vi "Main Page.vi"(8 "error in (no error)":errorcluster, 11 "Node Ptr":T1 format="%.0x") -> (0 "error out":errorcluster)   [LabVIEW 2016, in "UDP Sender System Explorer.lvlib"]
uses:
  UDP Sender System Explorer.lvlib
  <vilib>/NI Veristand/Custom Device API/Custom Device Item Ref.ctl
  Shared/Constants.vi
  <vilib>/NI Veristand/Custom Device API/Get Item Property (String).vi
  <vilib>/NI Veristand/Custom Device API/Get Item Property (U16).vi
  <vilib>/NI Veristand/Custom Device API/Set Item Property (String).vi
  <vilib>/NI Veristand/Custom Device API/Set Item Property (U16).vi
  <vilib>/NI Veristand/Custom Device API/Custom Device API.lvlib
  Shared/UDP Sender Shared.lvlib
panel:
  out "Channels to Send":i32(listbox)
  in  "Destination Port":u16
  in  "Destination IP":string
  in  "Header":cluster{"Section Name":string}={"Section Name"="Custom Device Item Settings"}
  in  "Description":string
  in  "Name":string
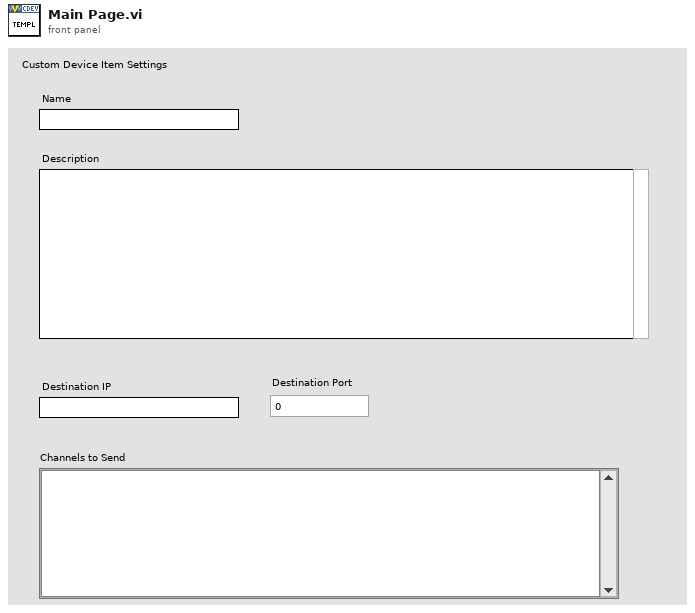
[diagram p1: front panel]
types:
  T1 = typedef "Custom Device API.lvlib/Custom Device Item Ref.ctl" = u64
  T2 = typedef "Custom Device API.lvlib/Custom Device Item Info.ctl" = cluster{"Name":string, "Is Channel":bool, "GUID":string, "Is Waveform":bool}
  T3 = typedef "Custom Device API.lvlib/Custom Device Commands.ctl" = enum16{"Default", "Item renamed", "Shutdown", "Dynamic button pressed"}
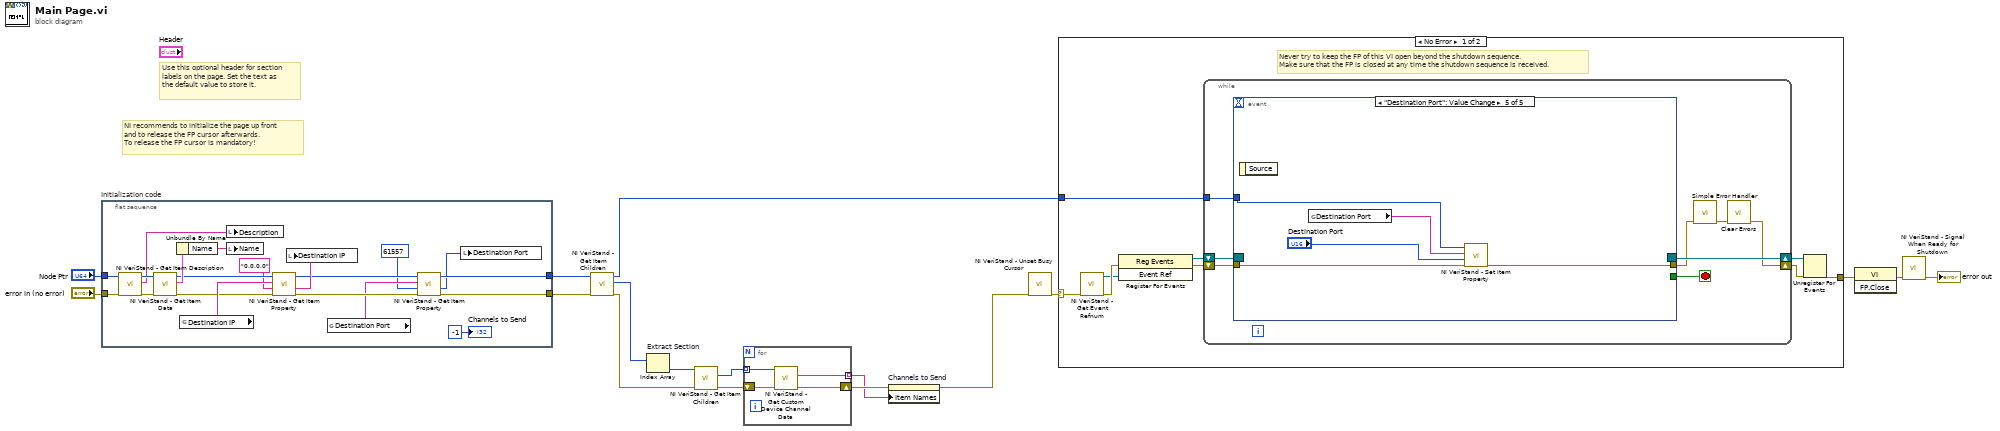
[diagram p0: block diagram]
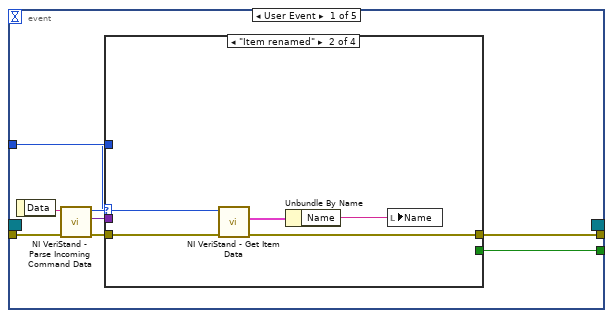
[diagram p2: hidden frame]
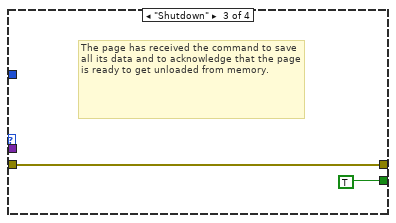
[diagram p4: hidden frame]
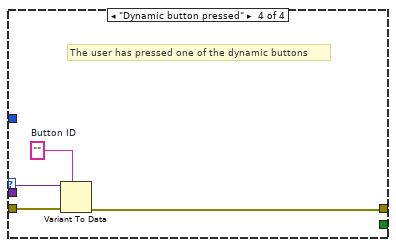
[diagram p5: hidden frame]
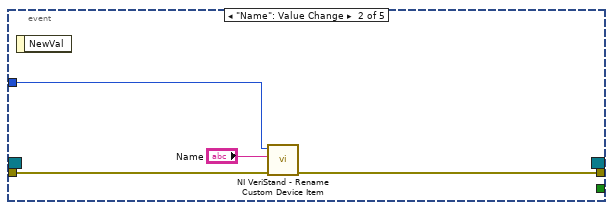
[diagram p6: hidden frame]
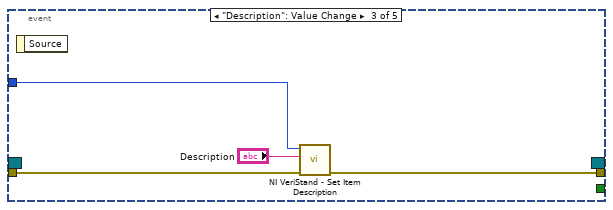
[diagram p7: hidden frame]
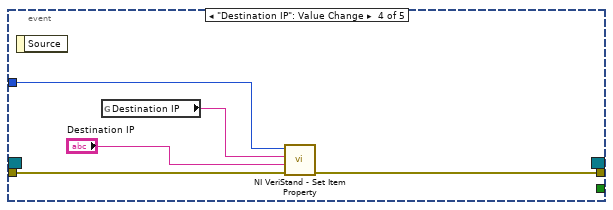
[diagram p8: hidden frame]
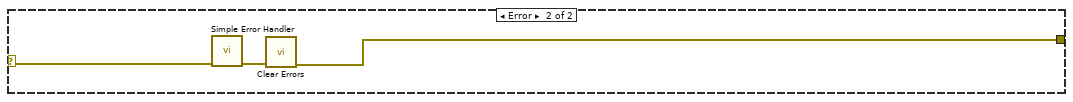
[diagram p9: hidden frame]
diagram:
  # "Use this optional header for section labels on the page. Set the text as the default value to store it."
  # "NI recommends to initialize the page up front\nand to release the FP cursor afterwards.\nTo release the FP cursor is mandatory!"
  n1 = flat-sequence "Initialization code" {
    tunnel: "error in (no error)" -> [w36]
    tunnel: "Node Ptr" -> [w35]
    tunnel: [w23] -> w2
    tunnel: [w22] -> w1
    frame #0 {
      n2 = call <vilib>:"NI VeriStand - Get Item Description.vi"("error in (no error)"=w36, "Item Ref in"=w35) -> ("error out"=w33:errorcluster, "Description"=w34:string, "Item Ref out"=w37:T1)  [unwired: 7 out]
      n3 = call <vilib>:"NI VeriStand - Get Item Data.vi"("error in (no error)"=w33, "Item Ref in"=w37) -> ("error out"=w27:errorcluster, "Item Info"=w32:T2, "Item Ref out"=w30:T1)  [unwired: 7 out]
      n4 = Unbundle By Name(w32) -> ("Name"=w31:string)
      n5 = global read "Constants.vi" "Destination IP"() -> (w29:string)
      n6 = local write "Description"(w34) -> ()
      n7 = local write "Name"(w31) -> ()
      n8 = call-poly <vilib>:"NI VeriStand - Get Item Property.vi"("error in (no error)"=w27, "Default Value"="0.0.0.0", "Property Name"=w29, "Item Ref in"=w30) -> ("error out"=w24:errorcluster, "Value"=w26:string, "Item Ref out"=w25:T1)  [unwired: 4 in, 1 out]
      n9 = local write "Destination IP"(w26) -> ()
      n10 = global read "Constants.vi" "Destination Port"() -> (w21:string)
      n11 = call-poly <vilib>:"NI VeriStand - Get Item Property.vi"("error in (no error)"=w24, "Default Value"=u16 61557, "Property Name"=w21, "Item Ref in"=w25) -> ("error out"=w23:errorcluster, "Value"=w19:u16, "Item Ref out"=w22:T1)  [unwired: 4 in, 1 out]
      n12 = local write "Destination Port"(w19) -> ()
      "Channels to Send" <- -1 ("Channels to Send")
    }
  }
  n13 = call <vilib>:"NI VeriStand - Get Item Children.vi"("error in (no error)"=w2, "Item Ref in"=w1) -> ("error out"=w8:errorcluster, "Child Refs"=w10:T1[], "Item Ref out"=w11:T1)  [unwired: 6 in, 1 out]
  n14 = Index Array "Extract Section"(array=w10) -> (element=w9:T1)  [unwired: 1 in]
  n15 = call <vilib>:"NI VeriStand - Get Item Children.vi"("error in (no error)"=w8, "Item Ref in"=w9) -> ("error out"=w6:errorcluster, "Child Refs"=w7:T1[])  [unwired: 6 in, 2 out]
  n16 = for {
    tunnel: w7 -> [w41] mode=indexing
    shift-right: [w39] -> w5
    shift-left: w6 -> [w40]
    tunnel: [w38] -> w4 mode=indexing
    n17 = call <vilib>:"NI VeriStand - Get Custom Device Channel Data.vi"("error in (no error)"=w40, "Channel Ref in"=w41) -> ("error out"=w39:errorcluster, "Channel Name"=w38:string)  [unwired: 4 in, 4 out]
  }
  n18 = property on="Channels to Send" class="LstBox (strict)"(error in=w5, "Item Names"=w4) -> (error out=w3:errorcluster)  [unwired: 1 in, 1 out]
  n19 = call <vilib>:"NI VeriStand - Unset Busy Cursor.vi"("error in (no error)"=w3) -> ("error out"=w13:errorcluster)  [unwired: 10 out]
  n20 = case shown="No Error" w13 {
    selector: w13 -> [w42 w99]
    tunnel: [w47 w97] -> w17
    tunnel: w11 -> [w43 _]
    frame No Error {
      # "Never try to keep the FP of this VI open beyond the shutdown sequence.\nMake sure that the FP is closed at any time the shutdown sequence is received."
      n21 = call <vilib>:"NI VeriStand - Get Event Refnum.vi"("error in (no error)"=w42) -> ("error out"=w50:errorcluster, "Event Ref"=w46:refnum<user-event>)  [unwired: 9 out]
      n22 = register-events(error in=w50, w46) -> (reference out=w44:refnum<event-registration>, error out=w45:errorcluster)  [unwired: 1 in]
      n23 = while {
        tunnel: w43 -> [w54]
        shift-right: [w51] -> w48
        shift-left: w45 -> [w57]
        shift-right: [w58] -> w49
        shift-left: w44 -> [w56]
        stop <- w55 stop-if-true
        n24 = event shown="[4] \"Destination Port\": Value Change" {
          selector: w56 -> [_ _ _ _ _]
          dyn-events: [_ _ _ _ _] -> w58
          timeout: _ -> [_ _ _ _ _]
          tunnel: w57 -> [w66 w82 w85 w90 w94]
          tunnel: [w62 _ _ _ _] -> w55
          tunnel: [w61 w81 w84 w89 w93] -> w53
          tunnel: w54 -> [w60 w80 w86 w91 w96]
          event User Event {
            n25 = event-data() -> ("Data"=w65:string)  [unwired: 1 out]
            n26 = call <vilib>:"NI VeriStand - Parse Incoming Command Data.vi"("error in (no error)"=w66, "Incoming data"=w65) -> ("error out"=w64:errorcluster, "Outgoing data"=w59:variant, "Action"=w63:T3)  [unwired: 7 out]
            n27 = case shown="\"Item renamed\"" w63 {
              tunnel: w64 -> [w67 w72 w73 w78]
              tunnel: [_ _ TRUE _] -> w62
              tunnel: [w67 w69 w73 w75] -> w61
              tunnel: w60 -> [_ w71 _ _]
              tunnel: w59 -> [_ _ _ w77]
              frame "Default", Default {
              }
              frame "Item renamed" {
                n28 = call <vilib>:"NI VeriStand - Get Item Data.vi"("error in (no error)"=w72, "Item Ref in"=w71) -> ("error out"=w69:errorcluster, "Item Info"=w70:T2)  [unwired: 8 out]
                n29 = Unbundle By Name(w70) -> ("Name"=w68:string)
                n30 = local write "Name"(w68) -> ()
              }
              frame "Shutdown" {
                # "The page has received the command to save all its data and to acknowledge that the page is ready to get unloaded from memory."
              }
              frame "Dynamic button pressed" {
                w76 = ""  # Button ID
                # "The user has pressed one of the dynamic buttons"
                n31 = Variant To Data(error in=w78, type=w76, Variant=w77) -> (error out=w75:errorcluster)  [unwired: 1 out]
              }
            }
          }
          event "Name": Value Change {
            n32 = event-data() -> ()  [unwired: 2 out]
            n33 = call <vilib>:"NI VeriStand - Rename Custom Device Item.vi"("error in (no error)"=w82, "New Name"="Name", "Item Ref in"=w80) -> ("error out"=w81:errorcluster)  [unwired: 1 in, 7 out]
          }
          event "Description": Value Change {
            n34 = event-data() -> ()  [unwired: 2 out]
            n35 = call <vilib>:"NI VeriStand - Set Item Description.vi"("error in (no error)"=w85, "Description"="Description", "Item Ref in"=w86) -> ("error out"=w84:errorcluster)  [unwired: 8 out]
          }
          event "Destination IP": Value Change {
            n36 = event-data() -> ()  [unwired: 2 out]
            n37 = global read "Constants.vi" "Destination IP"() -> (w87:string)
            n38 = call-poly <vilib>:"NI VeriStand - Set Item Property.vi"("error in (no error)"=w90, "Value"="Destination IP", "Property Name"=w87, "Item Ref in"=w91) -> ("error out"=w89:errorcluster)  [unwired: 5 in, 2 out]
          }
          event "Destination Port": Value Change {
            n39 = event-data() -> ()  [unwired: 2 out]
            n40 = global read "Constants.vi" "Destination Port"() -> (w92:string)
            n41 = call-poly <vilib>:"NI VeriStand - Set Item Property.vi"("error in (no error)"=w94, "Value"="Destination Port", "Property Name"=w92, "Item Ref in"=w96) -> ("error out"=w93:errorcluster)  [unwired: 5 in, 2 out]
          }
        }
        n42 = call <vilib>:"Simple Error Handler.vi"("error in (no error)"=w53) -> ("error out"=w52:errorcluster)  [unwired: 1 in, 7 out]
        n43 = call <vilib>:"Clear Errors.vi"("error in (no error)"=w52) -> ("error out"=w51:errorcluster)  [unwired: 1 in, 5 out]
      }
      n44 = Unregister For Events(event registration refnum=w49, error in=w48) -> (error out=w47:errorcluster)
    }
    frame Error {
      n45 = call <vilib>:"Simple Error Handler.vi"("error in (no error)"=w99) -> ("error out"=w98:errorcluster)  [unwired: 1 in, 7 out]
      n46 = call <vilib>:"Clear Errors.vi"("error in (no error)"=w98) -> ("error out"=w97:errorcluster)  [unwired: 1 in, 5 out]
    }
  }
  n47 = invoke class="VI" method="FP.Close"(error in=w17) -> (error out=w16:errorcluster)  [unwired: 2 in, 2 out]
  n48 = call <vilib>:"NI VeriStand - Signal When Ready for Shutdown.vi"("error in (no error)"=w16) -> ("error out"=→"error out":errorcluster)  [unwired: 10 out]
